vi "Control, Get Corner.vi"(6 "error in":errorcluster, 9 "Ctl ref":refnum<vi>) -> (0 "error out":errorcluster, 1 "bottom":i32, 2 "right":i32, 3 "Ctl ref dup":refnum<vi>)   [LabVIEW 2010]
doc: "This function gets a GUI control's lower right corner pane coordinates relative to the origin."
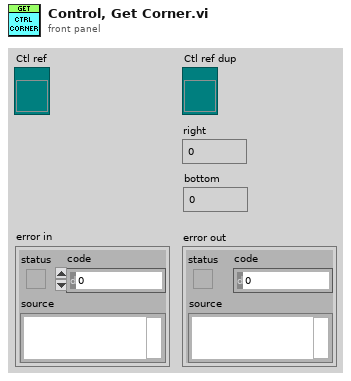
[diagram p1: front panel]
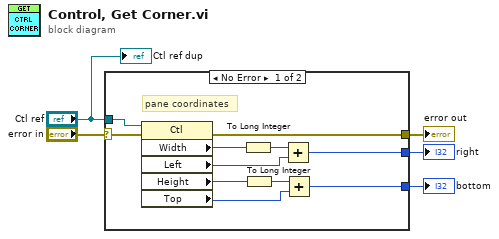
[diagram p0: block diagram]
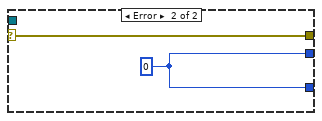
[diagram p2: hidden frame]
diagram:
  n1 = case shown="No Error" "error in" {
    selector: "error in" -> [w15 w18]
    tunnel: [w10 w18] -> w5
    tunnel: "Ctl ref" -> [w16 _]
    tunnel: [w7 w17] -> w2
    tunnel: [w6 w17] -> w1
    frame No Error {
      # "pane coordinates"
      n2 = property class="Ctl"(reference=w16, error in=w15) -> (error out=w10:errorcluster, "Width"=w14:u32, "Left"=w9:i32, "Height"=w11:u32, "Top"=w8:i32)  [unwired: 1 out]
      n3 = To Long Integer(number=w14) -> (32bit integer=w13:i32)
      n4 = To Long Integer(number=w11) -> (32bit integer=w12:i32)
      n5 = Add(x=w13, y=w9) -> (x+y=w7:i32)
      n6 = Add(x=w12, y=w8) -> (x+y=w6:i32)
    }
    frame Error {
      w17 = 0 ("Left")
    }
  }
  "error out" <- w5
  "right" <- w2
  "bottom" <- w1
  "Ctl ref dup" <- "Ctl ref"
